vi "QuadRotor_Monitoring_LV3_NODistanceMeasure.vi"() -> ()   [LabVIEW 2015]
uses:
  <vilib>/Instr/_visa.llb/VISA Set IO Buffer Mask.ctl
  <vilib>/Instr/_visa.llb/VISA Configure Serial Port (Instr).vi
panel:
  out "GPS_Speed_Gaud":ext(knob) scale=0.0..100.0
  out "GPS_LON_TRANSPORT":ext format="%#.7f"
  out "GPS_LAT_TRANSPORT":ext format="%#.7f"
  out "GPS_LON_HOME":ext format="%#.7f"
  out "GPS_LAT_HOME":ext format="%#.7f"
  out "MotorBackRf":dbl(slide) scale=1000.0..2000.0
  out "MotorBackLf":dbl(slide) scale=1000.0..2000.0
  out "MotorFrontRf":dbl(slide) scale=1000.0..2000.0
  out "MotorFrontLf":dbl(slide) scale=1000.0..2000.0
  in  "Lontitude_Transport":i32=1001113510
  in  "Latitude_Transport":i32=20030062
  in  "Lon_home":i32=1001110710
  in  "Lat_home":i32=20029288
  out "(GPS_numSat)":u16(slide) scale=0.0..20.0
  out "return count 2":u32
  out "Roob":i32
  out "Altitude_(Auto)":ext format="%#_3g"
  in  "Set_Altitude_(Auto)":dbl=12.0
  out "string":string
  out "Mode":ext format="%.2f"
  out "Altitude":dbl(slide) scale=0.0..20.0
  out "Altitude":ext format="%.2f"
  out "Yaw":dbl(knob) scale=-180.0..180.0
  out "Pitch":dbl(knob) scale=-90.0..90.0
  out "Roll":dbl(knob) scale=-90.0..90.0
  in  "Write to Quad":bool
  out "Header_58":u8
  out "GPS_LONGTITUDE":ext format="%#.7f"
  out "GPS_LATTITUDE":ext format="%#.7f"
  out "return count":u32
  in  "stop":bool
  in  "VISA Serial Data":refnum<visa-resource-name>
  # "Quad Rotor Monitoring and Control with GPS Waypoint"
  # "Data Write to Autonomous Quad Rotor (LAT 9 Point), (LON 10 Point) with Google Map tracking Navigator"
  # "Ex  13.8591411 = 138591411 , 100.5231704 = 1005231704 Using in integer  I32"
  # "9 Point"
  # "10 Point"
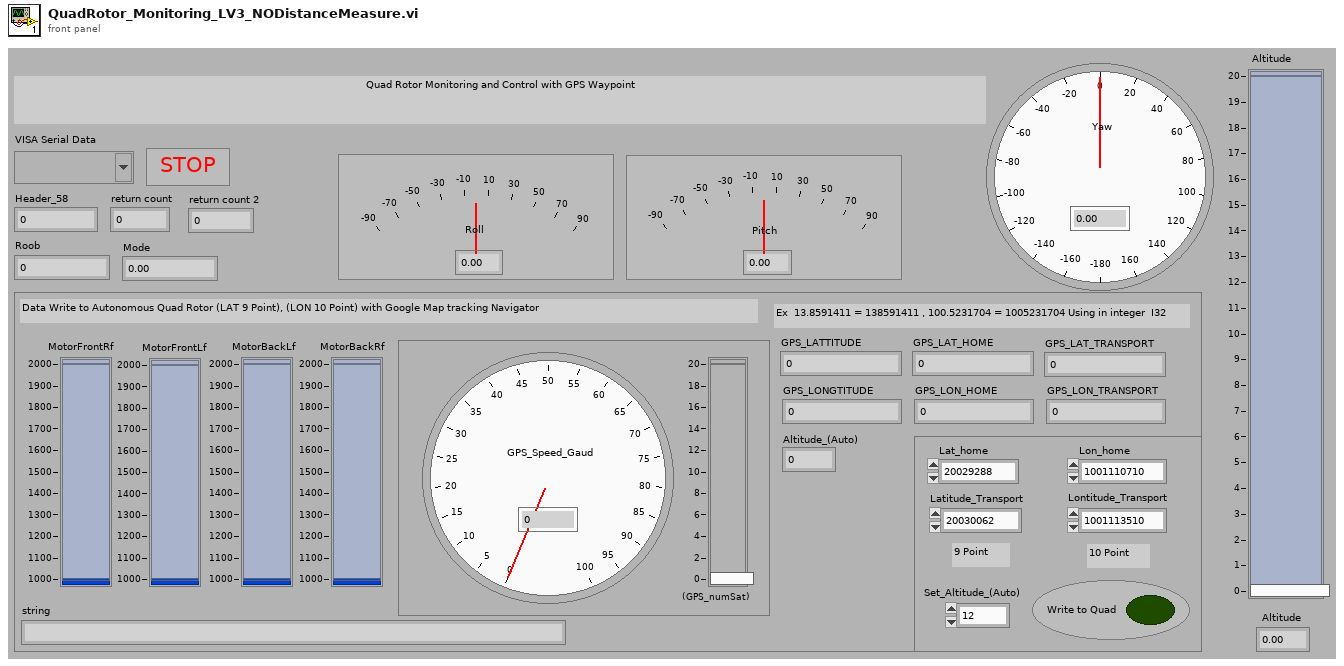
[diagram p1: front panel]
types:
  T1 = typedef "VISA Set IO Buffer Mask.ctl" = u16
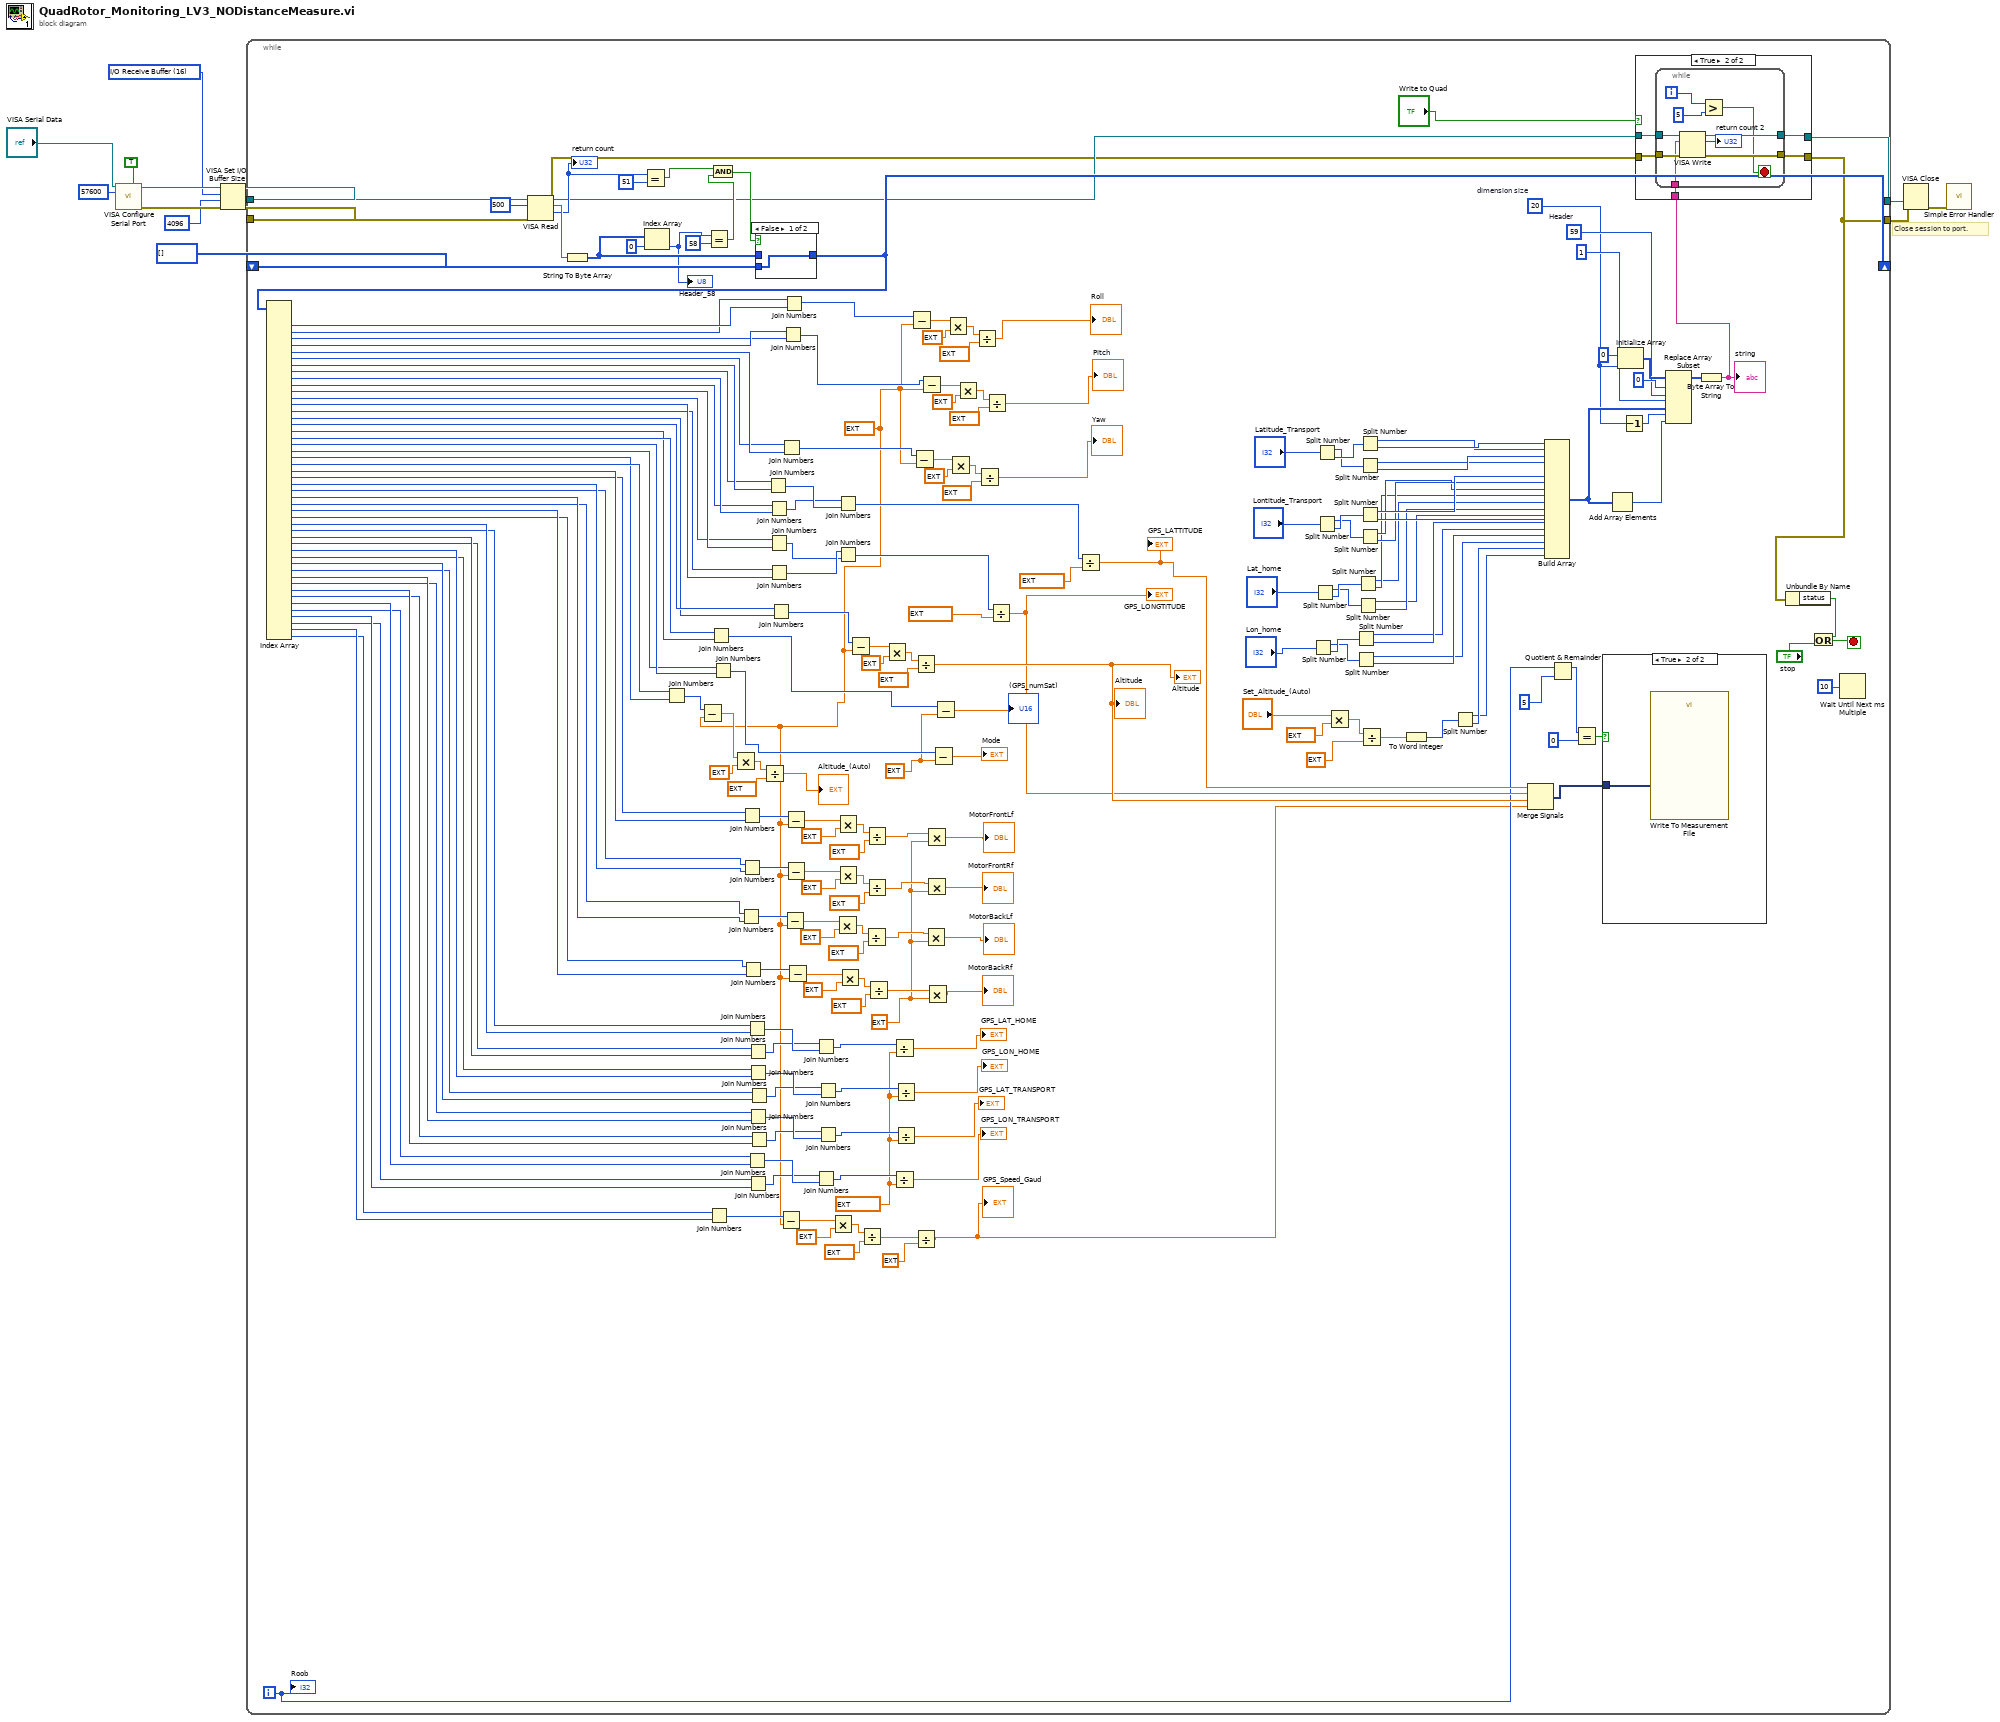
[diagram p0: block diagram]
diagram:
  w10 = T1 16 items=["I/O Receive Buffer"=16, "I/O Transmit Buffer"=32, "I/O Receive and Transmit Buffer"=48] ("Mask")
  # "Close session to port."
  n1 = call-poly "VISA Configure Serial Port"("VISA resource name"="VISA Serial Data", "Enable Termination\nChar (T)"=TRUE ("Enable Termination\nChar (T)"), "baud rate (9600)"=u32 57600) -> ("VISA resource name out"=w12:refnum<visa-resource-name>, "error out"=w11:errorcluster)  [unwired: 7 in, 4 out]
  n2 = VISA Set I/O Buffer Size(VISA resource name=w12, mask (16)=w10, size (4096)=u32 4096, error in (no error)=w11) -> (VISA resource name out=w8:refnum<visa-resource-name>, error out=w6:errorcluster)
  n3 = while {
    tunnel: [w194] -> w7
    tunnel: w8 -> [w235]
    tunnel: [w193] -> w5
    tunnel: w6 -> [w234]
    shift-right: [w204] -> _
    shift-left: u8[] [] ("unsigned byte array") -> [w205]
    i -> [w100]
    stop <- w238 stop-if-true
    w41 = ext 10000000.0 ("y")
    w60 = ext 10.0 ("y")
    w115 = 20  # dimension size
    w162 = u8 59  # Header
    w107 = ext 255.0 ("y")
    w17 = ext 32767.0 ("y")
    n4 = VISA Read(VISA resource name=w235, byte count=u32 500, error in (no error)=w234) -> (VISA resource name out=w196:refnum<visa-resource-name>, read buffer=w208:string, return count=w201:u32, error out=w195:errorcluster)
    "return count" <- w201
    n5 = String To Byte Array(string=w208) -> (unsigned byte array=w206:u8[])
    n6 = Equal?(x=w201, y=u32 51) -> (x = y?=w199:bool)
    n7 = Index Array(array=w206, index=0) -> (element=w198:u8)
    "Header_58" <- w198
    n8 = Equal?(x=w198, y=u8 58) -> (x = y?=w203:bool)
    n9 = And(x=w199, y=w203) -> (x .and. y?=w202:bool)
    n10 = case shown="False" w202 {
      tunnel: w206 -> [_ w257]
      tunnel: [w256 w257] -> w204
      tunnel: w205 -> [w256 _]
      frame False {
      }
      frame True {
      }
    }
    n11 = Index Array(array=w204) -> (element #2=w228:u8, element #3=w227:u8, element #4=w225:u8, element #5=w226:u8, element #6=w232:u8, element #7=w231:u8, element #8=w230:u8, element #9=w229:u8, element #10=w189:u8, element #11=w188:u8, element #12=w185:u8, element #13=w184:u8, element #14=w183:u8, element #15=w182:u8, element #16=w173:u8, element #17=w179:u8, element #18=w171:u8, element #19=w172:u8, element #20=w170:u8, element #21=w169:u8, element #22=w126:u8, element #23=w127:u8, element #24=w76:u8, element #25=w75:u8, element #26=w74:u8, element #27=w73:u8, element #28=w72:u8, element #29=w71:u8, element #30=w70:u8, element #31=w69:u8, element #32=w35:u8, element #33=w34:u8, element #34=w33:u8, element #35=w32:u8, element #36=w31:u8, element #37=w30:u8, element #38=w29:u8, element #39=w28:u8, element #40=w27:u8, element #41=w26:u8, element #42=w25:u8, element #43=w24:u8, element #44=w23:u8, element #45=w22:u8, element #46=w21:u8, element #47=w20:u8, element #48=w19:u8, element #49=w18:u8)  [unwired: 49 in, 1 out]
    n12 = Join Numbers(hi=w127, lo=w126) -> ((hi.lo)=w125:u16)
    n13 = Subtract(x=w125, y=w17) -> (x-y=w121:ext)
    n14 = Join Numbers(hi=w18, lo=w19) -> ((hi.lo)=w36:u16)
    n15 = Join Numbers(hi=w172, lo=w171) -> ((hi.lo)=w106:u16)
    n16 = Join Numbers(hi=w169, lo=w170) -> ((hi.lo)=w110:u16)
    n17 = Multiply(x=w121, y=ext 100.0) -> (x*y=w123:ext)
    n18 = Join Numbers(hi=w71, lo=w72) -> ((hi.lo)=w82:u16)
    n19 = Join Numbers(hi=w75, lo=w76) -> ((hi.lo)=w92:u16)
    n20 = Join Numbers(hi=w73, lo=w74) -> ((hi.lo)=w87:u16)
    n21 = Join Numbers(hi=w69, lo=w70) -> ((hi.lo)=w77:u16)
    n22 = Join Numbers(hi=w34, lo=w35) -> ((hi.lo)=w57:u16)
    n23 = Join Numbers(hi=w22, lo=w23) -> ((hi.lo)=w48:u16)
    n24 = Join Numbers(hi=w32, lo=w33) -> ((hi.lo)=w56:u16)
    n25 = Join Numbers(hi=w20, lo=w21) -> ((hi.lo)=w47:u16)
    n26 = Join Numbers(hi=w30, lo=w31) -> ((hi.lo)=w54:u16)
    n27 = Join Numbers(hi=w26, lo=w27) -> ((hi.lo)=w51:u16)
    n28 = Join Numbers(hi=w28, lo=w29) -> ((hi.lo)=w53:u16)
    n29 = Join Numbers(hi=w24, lo=w25) -> ((hi.lo)=w50:u16)
    n30 = Divide(x=w123, y=ext 32767.0) -> (x/y=→"Altitude_(Auto)":ext)
    n31 = Join Numbers(hi=w229, lo=w230) -> ((hi.lo)=w187:u16)
    n32 = Join Numbers(hi=w188, lo=w189) -> ((hi.lo)=w186:u16)
    n33 = Join Numbers(hi=w184, lo=w185) -> ((hi.lo)=w167:u16)
    n34 = Join Numbers(hi=w182, lo=w183) -> ((hi.lo)=w168:u16)
    n35 = Join Numbers(hi=w179, lo=w173) -> ((hi.lo)=w174:u16)
    n36 = Subtract(x=w36, y=w17) -> (x-y=w39:ext)
    n37 = Join Numbers(hi=w231, lo=w232) -> ((hi.lo)=w214:u16)
    n38 = Join Numbers(hi=w226, lo=w225) -> ((hi.lo)=w209:u16)
    n39 = Join Numbers(hi=w227, lo=w228) -> ((hi.lo)=w223:u16)
    n40 = Subtract(x=w82, y=w17) -> (x-y=w85:ext)
    n41 = Subtract(x=w92, y=w17) -> (x-y=w95:ext)
    n42 = Subtract(x=w87, y=w17) -> (x-y=w90:ext)
    n43 = Subtract(x=w77, y=w17) -> (x-y=w80:ext)
    n44 = Join Numbers(hi=w56, lo=w57) -> ((hi.lo)=w55:u32)
    n45 = Join Numbers(hi=w47, lo=w48) -> ((hi.lo)=w46:u32)
    n46 = Join Numbers(hi=w53, lo=w54) -> ((hi.lo)=w52:u32)
    n47 = Join Numbers(hi=w50, lo=w51) -> ((hi.lo)=w49:u32)
    n48 = Multiply(x=w39, y=ext 100.0) -> (x*y=w40:ext)
    n49 = Multiply(x=w85, y=ext 185.0) -> (x*y=w86:ext)
    n50 = Join Numbers(hi=w186, lo=w187) -> ((hi.lo)=w191:u32)
    n51 = Join Numbers(hi=w168, lo=w167) -> ((hi.lo)=w181:u32)
    n52 = Multiply(x=w95, y=ext 185.0) -> (x*y=w96:ext)
    n53 = Multiply(x=w90, y=ext 185.0) -> (x*y=w91:ext)
    n54 = Multiply(x=w80, y=ext 185.0) -> (x*y=w81:ext)
    n55 = Subtract(x=w174, y=w17) -> (x-y=w178:ext)
    n56 = Divide(x=w40, y=ext 32767.0) -> (x/y=w16:ext)
    n57 = Divide(x=w86, y=ext 32767.0) -> (x/y=w63:ext)
    n58 = Divide(x=w96, y=ext 32767.0) -> (x/y=w61:ext)
    n59 = Divide(x=w91, y=ext 32767.0) -> (x/y=w62:ext)
    n60 = Divide(x=w81, y=ext 32767.0) -> (x/y=w68:ext)
    n61 = Multiply(x=w178, y=ext 100.0) -> (x*y=w176:ext)
    n62 = Divide(x=w55, y=w41) -> (x/y=→"GPS_LAT_HOME":ext)
    n63 = Divide(x=w46, y=w41) -> (x/y=→"GPS_LON_TRANSPORT":ext)
    n64 = Divide(x=w52, y=w41) -> (x/y=→"GPS_LON_HOME":ext)
    n65 = Divide(x=w49, y=w41) -> (x/y=→"GPS_LAT_TRANSPORT":ext)
    n66 = Subtract(x=w223, y=w17) -> (x-y=w222:ext)
    n67 = Subtract(x=w214, y=w17) -> (x-y=w218:ext)
    n68 = Divide(x=w176, y=ext 32767.0) -> (x/y=w105:ext)
    "Altitude" <- w105
    "Altitude" <- w105
    n69 = Divide(x=w16, y=ext 10.0) -> (x/y=w15:ext)
    "GPS_Speed_Gaud" <- w15
    n70 = Subtract(x=w209, y=w17) -> (x-y=w213:ext)
    n71 = Multiply(x=w63, y=w60) -> (x*y=→"MotorBackLf":ext)
    n72 = Multiply(x=w61, y=w60) -> (x*y=→"MotorFrontLf":ext)
    n73 = Multiply(x=w62, y=w60) -> (x*y=→"MotorFrontRf":ext)
    n74 = Multiply(x=w68, y=w60) -> (x*y=→"MotorBackRf":ext)
    n75 = Subtract(x=w110, y=w107) -> (x-y=→"Mode":ext)
    n76 = Subtract(x=w106, y=w107) -> (x-y=→"(GPS_numSat)":ext)
    n77 = Multiply(x=w222, y=ext 180.0) -> (x*y=w220:ext)
    n78 = Multiply(x=w218, y=ext 180.0) -> (x*y=w216:ext)
    n79 = Multiply(x=w213, y=ext 180.0) -> (x*y=w211:ext)
    n80 = Divide(x=w220, y=ext 32767.0) -> (x/y=→"Roll":ext)
    n81 = Divide(x=w216, y=ext 32767.0) -> (x/y=→"Yaw":ext)
    n82 = Divide(x=w211, y=ext 32767.0) -> (x/y=→"Pitch":ext)
    n83 = Divide(x=w181, y=ext 10000000.0) -> (x/y=w104:ext)
    "GPS_LONGTITUDE" <- w104
    n84 = Divide(x=w191, y=ext 10000000.0) -> (x/y=w103:ext)
    "GPS_LATTITUDE" <- w103
    n85 = Split Number(x="Lon_home") -> (hi(x)=w155:u16, lo(x)=w156:u16)
    n86 = Split Number(x="Lat_home") -> (hi(x)=w157:u16, lo(x)=w158:u16)
    n87 = Split Number(x="Lontitude_Transport") -> (hi(x)=w159:u16, lo(x)=w160:u16)
    n88 = Split Number(x="Latitude_Transport") -> (hi(x)=w137:u16, lo(x)=w138:u16)
    n89 = Multiply(x="Set_Altitude_(Auto)", y=ext 32767.0) -> (x*y=w130:ext)
    n90 = Split Number(x=w156) -> (hi(x)=w141:u8, lo(x)=w142:u8)
    n91 = Split Number(x=w155) -> (hi(x)=w139:u8, lo(x)=w140:u8)
    n92 = Split Number(x=w158) -> (hi(x)=w145:u8, lo(x)=w146:u8)
    n93 = Split Number(x=w157) -> (hi(x)=w143:u8, lo(x)=w144:u8)
    n94 = Split Number(x=w160) -> (hi(x)=w149:u8, lo(x)=w150:u8)
    n95 = Split Number(x=w159) -> (hi(x)=w147:u8, lo(x)=w148:u8)
    n96 = Split Number(x=w138) -> (hi(x)=w153:u8, lo(x)=w154:u8)
    n97 = Split Number(x=w137) -> (hi(x)=w151:u8, lo(x)=w152:u8)
    n98 = Divide(x=w130, y=ext 100.0) -> (x/y=w128:ext)
    n99 = To Word Integer(number=w128) -> (16bit integer=w131:i16)
    n100 = Split Number(x=w131) -> (hi(x)=w132:u8, lo(x)=w133:u8)
    n101 = Merge Signals(w103, w104, w105, w15) -> (w102:dynamicdata)
    n102 = Build Array(w154, w153, w152, w151, w150, w149, w148, w147, w146, w145, w144, w143, w142, w141, w140, w139, w133, w132) -> (w118:u8[])
    n103 = Quotient & Remainder(x=w100, y=u32 5) -> (x-y*floor(x/y)=w97:u32)  [unwired: 1 out]
    n104 = Equal?(x=w97, y=u32 0) -> (x = y?=w99:bool)
    n105 = case shown="True" w99 {
      tunnel: w102 -> [_ w239]
      frame False {
      }
      frame True {
        n106 = call "Write To Measurement File"("Signals"=w239) -> ()  [unwired: 16 in, 3 out]
      }
    }
    n107 = Add Array Elements(numeric array=w118) -> (sum=w117:u8)
    n108 = Initialize Array(u8 0, w115) -> (w166:u8[])
    n109 = Decrement(x=w115) -> (x-1=w116:i32)
    n110 = Replace Array Subset(array=w166, new element #1=w162, index #1=0 ("index"), new element #2=w118, index #2=1 ("index"), new element #3=w117, index #3=w116) -> (w161:u8[])
    n111 = Byte Array To String(unsigned byte array=w161) -> (string=w136:string)
    "string" <- w136
    n112 = case shown="True" "Write to Quad" {
      tunnel: w196 -> [w240 w246]
      tunnel: w195 -> [w241 w243]
      tunnel: [w240 w245] -> w194
      tunnel: [w241 w244] -> w193
      tunnel: w136 -> [_ w242]
      frame False {
      }
      frame True {
        n113 = while {
          tunnel: w246 -> [w255]
          tunnel: [w254] -> w245
          tunnel: [w253] -> w244
          tunnel: w243 -> [w252]
          tunnel: w242 -> [w251]
          i -> [w249]
          stop <- w247 stop-if-true
          n114 = VISA Write(VISA resource name=w255, write buffer=w251, error in (no error)=w252) -> (VISA resource name out=w254:refnum<visa-resource-name>, return count=→"return count 2":u32, error out=w253:errorcluster)
          n115 = Greater?(x=w249, y=5) -> (0:w247:bool)
        }
      }
    }
    n116 = Unbundle By Name(w193) -> ("status"=w236:bool)
    n117 = Or(x=w236, y="stop") -> (x .or. y?=w238:bool)
    n118 = Wait Until Next ms Multiple(millisecond multiple=u32 10) -> ()  [unwired: 1 out]
    "Roob" <- w100
  }
  n119 = VISA Close(VISA resource name=w7, error in (no error)=w5) -> (error out=w9:errorcluster)
  n120 = call <vilib>:"Simple Error Handler.vi"("error in (no error)"=w9) -> ()  [unwired: 1 in, 8 out]
